vi "Proyecto Intengrador Torres_Galora_Granda.vi"() -> ()   [LabVIEW 2026]
uses:
  <vilib>/MakerHub/LINX/Public/Peripherals/Analog/Analog Read 1 Chan.vi
  <vilib>/MakerHub/LINX/Public/Peripherals/Digital/Digital Write 1 Chan.vi
  <vilib>/MakerHub/LINX/Public/Peripherals/Analog/Analog Read N Chans.vi
  <vilib>/MakerHub/LINX/Public/Peripherals/Digital/Digital Write N Chans.vi
  <vilib>/MakerHub/LINX/Private/Local IO/LinxAnalogRead.vi
  <vilib>/MakerHub/LINX/Public/Utilities/Check Channel.vi
  <vilib>/MakerHub/LINX/Private/Local IO/LinxDigitalWrite.vi
  <vilib>/MakerHub/LINX/Public/Utilities/Open Serial.vi
  <vilib>/MakerHub/LINX/Private/Utilties/Generate Error.vi
  <vilib>/express/express shared/transition.llb/Dynamic To Waveform Array.vi
  <vilib>/express/express signal manip/GetorSetDDTAttributes/Set DDT Attributes/SetT0.vi
  <vilib>/express/express signal manip/GetorSetDDTAttributes/Set DDT Attributes/sub Set StartTimeStamp.vi
  <vilib>/express/express shared/transition.llb/Waveform Array To Dynamic.vi
  <vilib>/express/express signal manip/GetorSetDDTAttributes/Set DDT Attributes/Set DDT Properties.xnode
  <vilib>/MakerHub/LINX/LMH-LINX.lvlib
  <vilib>/express/express signal manip/GetorSetDDTAttributes/Set DDT Attributes/Set DDT Attributes.lvlib
panel:
  out "Numeric 6":dbl
  out "Numeric 5":dbl
  out "Numeric 4":dbl
  out "Numeric 3":dbl
  out "Numeric 2":dbl
  out "Numeric":dbl
  in  "Serial Port":refnum<visa-resource-name>="N/A"
  out "PSI DE\n FRENADO":dbl(graph)
  out "RPMS DEL \nMOTOR":dbl(graph)
  out "MÁXIMO DE \nRPM":bool
  out "BATERIA \nBAJA 20%":bool
  out "BATERIA AL\n100%":bool
  out "HOT":bool
  out "COLD":bool
  out "CARGA DE \nBATERÍA":dbl(slide) scale=0.0..100.0
  out "PRESIÓN DE \n FRENADO":dbl(knob) scale=0.0..50.0
  out "Temp.\n  °F":dbl(slide) scale=0.0..120.0
  out "Temp. \n  °C":dbl(slide) scale=0.0..120.0
  out "Temp\n  .°K":dbl(slide) scale=0.0..500.0
  out "MOTOR \nRPMS":dbl(knob) scale=0.0..7000.0
  in  "stop":bool
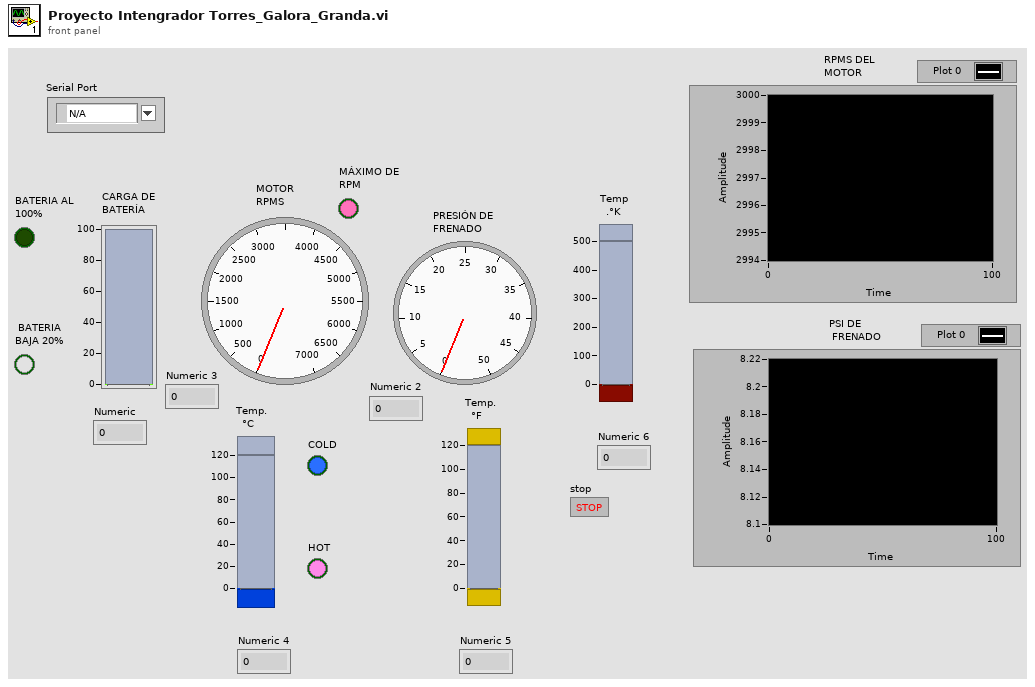
[diagram p1: front panel]
types:
  T1 = typedef "LMH-LINX.lvlib/LINX Ref.ctl" = cluster{"IO":T2, "Interface":T3, "LINX Device Config":T4}
  T2 = typedef "LMH-LINX.lvlib/Platform.ctl" = enum16{"Remote", "Local"}
  T3 = typedef "LMH-LINX.lvlib/Interface.ctl" = enum16{"Serial", "TCP"}
  T4 = typedef "LMH-LINX.lvlib/Device.lvlib/LINX Device Config.ctl" = cluster{"Interface":T3, "COM Port":refnum<visa-resource-name>, "TCP Configuration":T5, "Device Family":u8, "Device ID":u8, "Device Name":string, "TCP Ref":refnum<k5>, "Channels":T6}
  T5 = typedef "LMH-LINX.lvlib/Device.lvlib/TCP Config.ctl" = cluster{"IP Address":string, "Port":u16}
  T6 = typedef "LMH-LINX.lvlib/Channels.ctl" = cluster{"DI":u8[], "DO":u8[], "AI":u8[], "AO":u8[], "PWM":u8[], "QE":u8[], "UART":u8[], "I2C 2":u8[], "SPI":u8[], "CAN":u8[], "Servo":u8[], "AI Ref (V)":dbl, "AI Resolution (Bits)":u8, "AO Ref (V)":dbl, "AO Resolution (Bits)":u8}
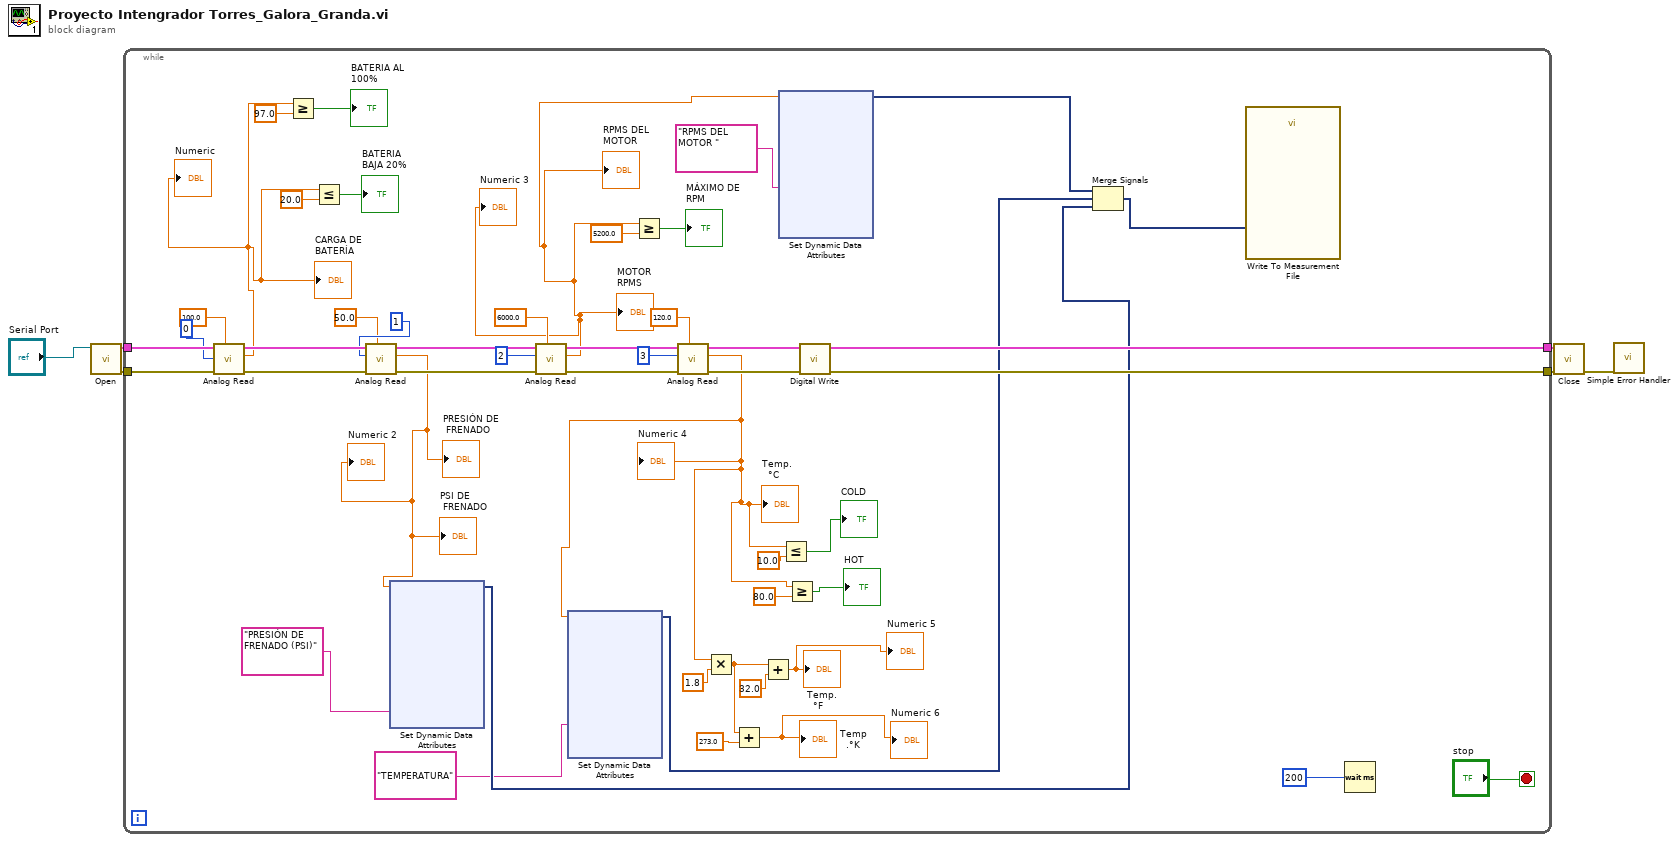
[diagram p0: block diagram]
diagram:
  n1 = call-poly <vilib>:"Open.vi"("Serial Port"="Serial Port") -> ("Error Out"=w3:errorcluster, "LINX Resource"=w6:T1)  [unwired: 8 in, 1 out]
  n2 = while {
    tunnel: w6 -> [w55]
    tunnel: [w27] -> w5
    tunnel: [w26] -> w4
    tunnel: w3 -> [w46]
    stop <- "stop" stop-if-true
    n3 = call-poly <vilib>:"Analog Read.vi"("Analog Ref Override (V)"=100.0, "Error In"=w46, "Analog Channel"=u8 0, "LINX Resource"=w55) -> ("Error Out"=w47:errorcluster, "Voltage"=w15:dbl, "LINX Resource"=w54:T1)  [unwired: 4 in, 1 out]
    "CARGA DE \nBATERÍA" <- w15
    "Numeric" <- w15
    n4 = Greater Or Equal?(x=w15, y=97.0) -> (x >= y?=→"BATERIA AL\n100%":bool)
    n5 = Less Or Equal?(x=w15, y=20.0) -> (x <= y?=→"BATERIA \nBAJA 20%":bool)
    n6 = call-poly <vilib>:"Analog Read.vi"("Analog Ref Override (V)"=50.0, "Error In"=w47, "Analog Channel"=u8 1, "LINX Resource"=w54) -> ("Error Out"=w48:errorcluster, "Voltage"=w14:dbl, "LINX Resource"=w53:T1)  [unwired: 4 in, 1 out]
    "PRESIÓN DE \n FRENADO" <- w14
    "PSI DE\n FRENADO" <- w14
    "Numeric 2" <- w14
    n7 = xnode "Set Dynamic Data Attributes"("Signal Name"="PRESIÓN DE FRENADO (PSI)", "Signals In"=w14) -> ("Signals Out"=w21:dynamicdata)  [unwired: 4 in, 1 out]
    n8 = call-poly <vilib>:"Analog Read.vi"("Analog Ref Override (V)"=6000.0, "Error In"=w48, "Analog Channel"=u8 2, "LINX Resource"=w53) -> ("Error Out"=w49:errorcluster, "Voltage"=w13:dbl, "LINX Resource"=w52:T1)  [unwired: 4 in, 1 out]
    "MOTOR \nRPMS" <- w13
    "RPMS DEL \nMOTOR" <- w13
    "Numeric 3" <- w13
    n9 = Greater Or Equal?(x=w13, y=5200.0) -> (x >= y?=→"MÁXIMO DE \nRPM":bool)
    n10 = call-poly <vilib>:"Analog Read.vi"("Analog Ref Override (V)"=120.0, "Error In"=w49, "Analog Channel"=u8 3, "LINX Resource"=w52) -> ("Error Out"=w50:errorcluster, "Voltage"=w12:dbl, "LINX Resource"=w51:T1)  [unwired: 4 in, 1 out]
    "Temp. \n  °C" <- w12
    "Numeric 4" <- w12
    n11 = xnode "Set Dynamic Data Attributes"("Signal Name"="TEMPERATURA", "Signals In"=w12) -> ("Signals Out"=w20:dynamicdata)  [unwired: 4 in, 1 out]
    n12 = Multiply(x=w12, y=1.8) -> (x*y=w41:dbl)
    n13 = Add(x=w41, y=273.0) -> (x+y=→"Temp\n  .°K" →"Numeric 6":dbl)
    n14 = Add(x=w41, y=32.0) -> (x+y=→"Temp.\n  °F" →"Numeric 5":dbl)
    n15 = xnode "Set Dynamic Data Attributes"("Signal Name"="RPMS DEL MOTOR ", "Signals In"=w13) -> ("Signals Out"=w22:dynamicdata)  [unwired: 4 in, 1 out]
    n16 = Less Or Equal?(x=w12, y=10.0) -> (x <= y?=→"COLD":bool)
    n17 = Greater Or Equal?(x=w12, y=80.0) -> (x >= y?=→"HOT":bool)
    n18 = call-poly <vilib>:"Digital Write.vi"("Error In"=w50, "LINX Resource"=w51) -> ("Error Out"=w26:errorcluster, "LINX Resource"=w27:T1)  [unwired: 8 in]
    n19 = Merge Signals(w22, w20, w21) -> (w23:dynamicdata)
    n20 = call "Write To Measurement File"("Signals"=w23) -> ()  [unwired: 16 in, 3 out]
    n21 = Wait (ms)(milliseconds to wait=u32 200) -> ()  [unwired: 1 out]
  }
  n22 = call <vilib>:"Close.vi"("Error In"=w4, "LINX Resource"=w5) -> ("Error Out"=w1:errorcluster)  [unwired: 9 in]
  n23 = call <vilib>:"Simple Error Handler.vi"("error in (no error)"=w1) -> ()  [unwired: 4 in, 5 out]
